vi "ViHandler.CheckForExistingVi.vi"(8 "error in (no error)":errorcluster, 9 "ViQueueName":string, 10 "ViReference":refnum<vi>, 11 "ViHandler in":refnum<class "ViHandler.lvclass">) -> (0 "error out":errorcluster, 1 "Found?":bool, 2 "ViInfo":T1, 3 "ViHandler out":refnum<class "ViHandler.lvclass">)   [LabVIEW 2016, in "ViHandler.lvclass"]
uses:
  ViHandler.lvclass
  ViHandler.ViInfo.ctl
  ViHandler.lvclass/ViHandler.ctl
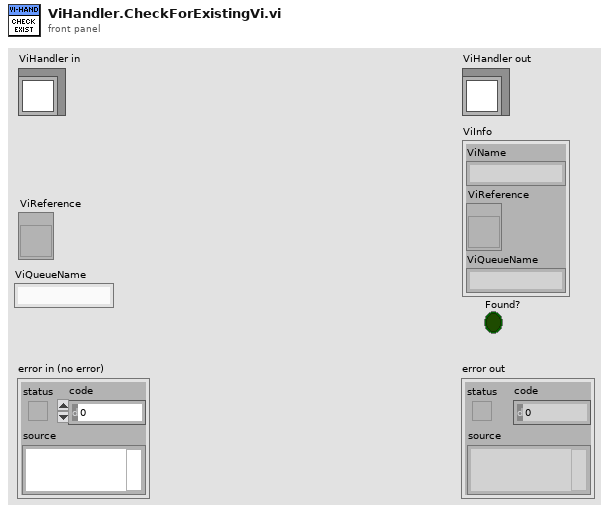
[diagram p1: front panel]
types:
  T1 = typedef "ViHandler.lvclass/ViHandler.ViInfo.ctl" = cluster{"ViName":string, "ViReference":refnum<vi>, "ViQueueName":string}
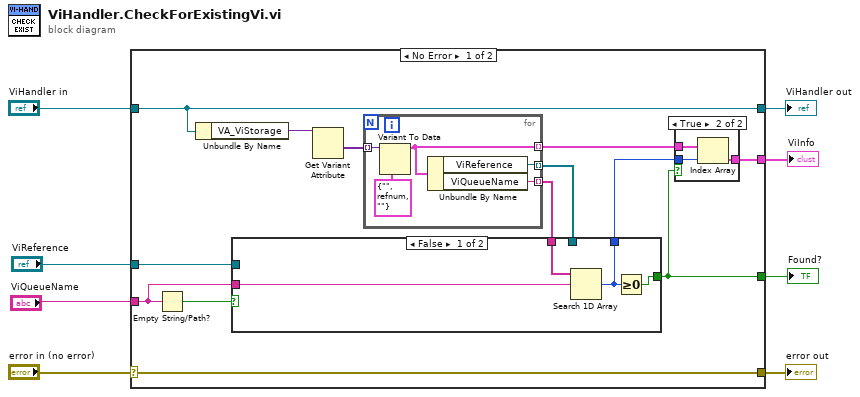
[diagram p0: block diagram]
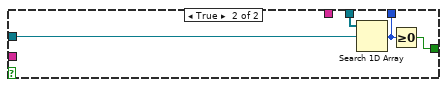
[diagram p3: hidden frame]
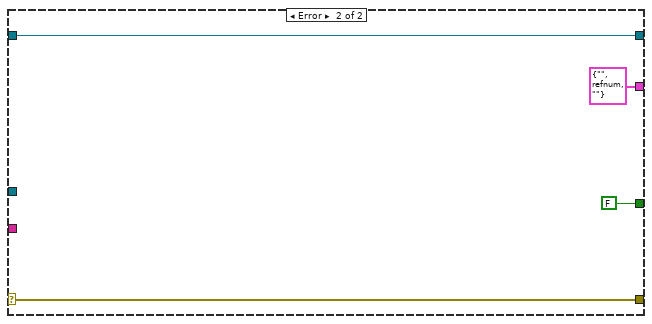
[diagram p4: hidden frame]
diagram:
  n1 = case shown="No Error" "error in (no error)" {
    selector: "error in (no error)" -> [w21 w41]
    tunnel: [w21 w41] -> w7
    tunnel: [w20 w40] -> w5
    tunnel: "ViHandler in" -> [w20 w40]
    tunnel: "ViQueueName" -> [w13 _]
    tunnel: "ViReference" -> [w16 _]
    tunnel: [w12 FALSE] -> w2
    tunnel: [w9 T1 {"ViName"="", "ViReference"=refnum, "ViQueueName"=""} ("ViInfo")] -> w1
    frame No Error {
      n2 = Empty String/Path?(string/path=w13) -> (empty?=w17:bool)
      n3 = Unbundle By Name(w20) -> ("VA_ViStorage"=w19:variant)
      n4 = Get Variant Attribute(Variant=w19) -> (values=w18:variant[])  [unwired: 3 in, 3 out]
      n5 = for {
        tunnel: w18 -> [w37] mode=indexing
        tunnel: [w35] -> w14 mode=indexing
        tunnel: [w34] -> w10 mode=indexing
        tunnel: [w33] -> w15 mode=indexing
        n6 = Variant To Data(type=T1 {"ViName"="", "ViReference"=refnum, "ViQueueName"=""} ("ViInfo"), Variant=w37) -> (data=w34:T1)  [unwired: 1 in, 1 out]
        n7 = Unbundle By Name(w34) -> ("ViReference"=w35:refnum<vi>, "ViQueueName"=w33:string)
      }
      n8 = case shown="False" w17 {
        tunnel: w16 -> [_ w31]
        tunnel: w15 -> [w28 _]
        tunnel: w14 -> [_ w32]
        tunnel: w13 -> [w27 _]
        tunnel: [w26 w30] -> w12
        tunnel: [w25 w29] -> w11
        frame False {
          n9 = Search 1D Array(1D array=w28, element=w27) -> (index of element=w25:i32)  [unwired: 1 in]
          n10 = Greater Or Equal To 0?(x=w25) -> (x >= 0?=w26:bool)
        }
        frame True {
          n11 = Search 1D Array(1D array=w32, element=w31) -> (index of element=w29:i32)  [unwired: 1 in]
          n12 = Greater Or Equal To 0?(x=w29) -> (x >= 0?=w30:bool)
        }
      }
      n13 = case shown="True" w12 {
        tunnel: w11 -> [_ w24]
        tunnel: w10 -> [_ w23]
        tunnel: [_ w22] -> w9
        frame False {
        }
        frame True {
          n14 = Index Array(array=w23, index=w24) -> (element=w22:T1)
        }
      }
    }
    frame Error {
    }
  }
  "error out" <- w7
  "ViHandler out" <- w5
  "Found?" <- w2
  "ViInfo" <- w1
